vi "Generate Core Library Errors File.vi"() -> ()   [LabVIEW 2020]
panel:
  out "All Files in Dir":path[](array[path])
  in  "project path":path
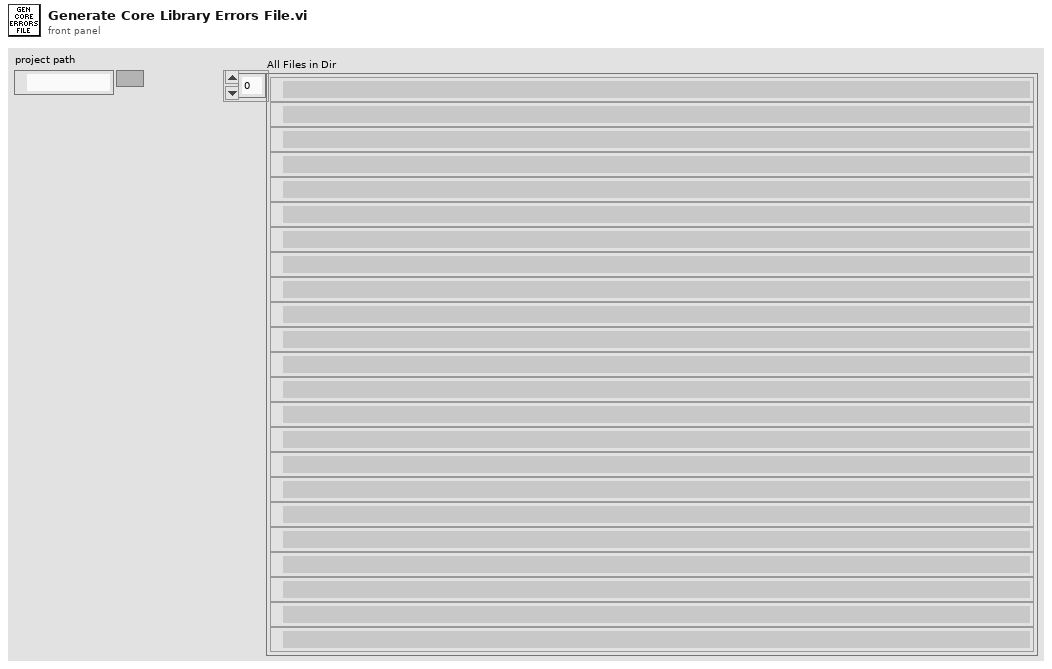
[diagram p1: front panel]
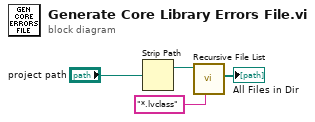
[diagram p0: block diagram]
diagram:
  n1 = Strip Path(path="project path") -> (stripped path=w3:path)  [unwired: 1 out]
  n2 = call <vilib>:"Recursive File List.vi"("pattern"="*.lvclass", "Folder Path"=w3) -> ("All Files in Dir"=→"All Files in Dir":path[])  [unwired: 5 in, 4 out]
